vi "Transmit Messages with Rate-based Schedule.vi"() -> ()   [LabVIEW 2023]
doc: "This program opens the specified card, builds a transmit schedule \nusing transmit interval information in the channel configuration file,\nand then transmits the messages with changing data."
uses:
  <instrlib>/BTICardLib/Private/Initialize By Card Number and Core Number.vi
  <instrlib>/BTICardLib/Private/Configure Core From XML.vi
  <instrlib>/BTI429Lib/Private/Tx/Configure/Configure Tx Channel From XML.vi
  <instrlib>/BTI429Lib/Private/Core/Action-Status/Start Channel.vi
  <instrlib>/BTI429Lib/Private/Utility/Get BNR Mantissa.vi
  <instrlib>/BTI429Lib/Private/Utility/Set BNR Mantissa.vi
  <instrlib>/BTI429Lib/Private/Core/Action-Status/Stop Channel.vi
  <instrlib>/BTICardLib/BTICardLV.lvlib
  <instrlib>/BTI429Lib/BTI429LV.lvlib
panel:
  out "Core Xml Path":path
  out "Channel Xml Path":path
  in  "Card number":i32
  in  "Channel number":i32
  in  "Core number":i32
  in  "Core Configuration XML file name":string="Core Config.xml"
  in  "Channel Configuration XML file name":string="Channel Config.xml"
  out "error out":errorcluster
  in  "stop":bool
  out "Data 1(MyLabel1)":u32 format="%.0b"
  out "Data 2(MyLabel2)":u32 format="%.0b"
  out "Data 3(MyLabel3)":u32 format="%.0b"
  # "ARINC 429: Transmit Messages with Rate-based Schedule"
  # "©2016 Astronics Ballard Technology"
  # "This program opens the specified card, builds a transmit schedule \nusing transmit interval information in the channel configuration file,\nand then transmits the messages with changing data."
  # "Always Stop the card\nand Close the card when\ndone. Otherwise, the hardware\ncontinues to operate."
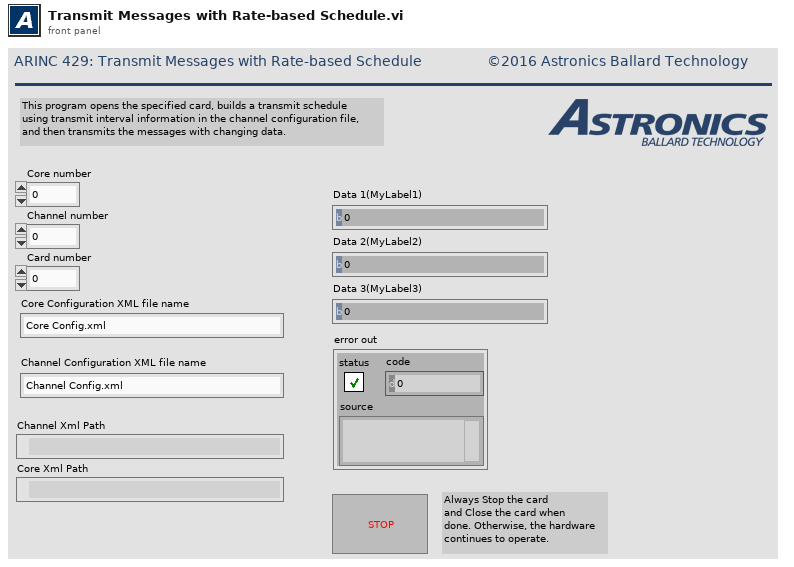
[diagram p1: front panel]
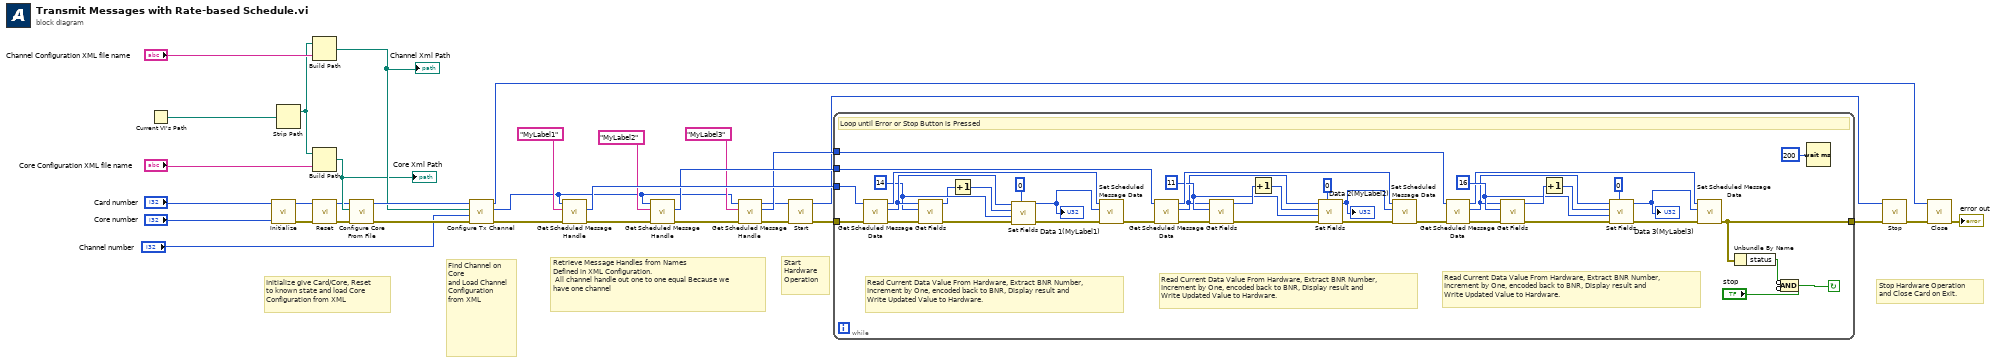
[diagram p0: block diagram]
diagram:
  # "Stop Hardware Operation\nand Close Card on Exit."
  # "Start Hardware\nOperation"
  # "Retrieve Message Handles from Names\nDefined in XML Configuration. \n All channel handle out one to one equal Because we have one channel"
  # "Find Channel on Core\nand Load Channel Configuration\nfrom XML"
  # "Initialize give Card/Core, Reset\nto known state and load Core\nConfiguration from XML"
  n1 = Current VI's Path() -> (path=w13:path)
  n2 = call-poly <instrlib>:"Initialize.vi"("core number"="Core number", "card number"="Card number") -> ("error out"=w6:errorcluster, "core handle out"=w7:u64)  [unwired: 8 in]
  n3 = Strip Path(path=w13) -> (stripped path=w10:path)  [unwired: 1 out]
  n4 = Build Path(base path=w10, name or relative path="Channel Configuration XML file name") -> (appended path=w12:path)
  "Channel Xml Path" <- w12
  n5 = Build Path(base path=w10, name or relative path="Core Configuration XML file name") -> (appended path=w8:path)
  "Core Xml Path" <- w8
  n6 = call <instrlib>:"Reset.vi"("error in (no error)"=w6, "core handle in"=w7) -> ("error out"=w4:errorcluster, "core handle out"=w5:u64)  [unwired: 8 in]
  n7 = call-poly <instrlib>:"Configure Core From File.vi"("error in (no error)"=w4, "configuration file path"=w8, "core handle in"=w5) -> ("error out"=w19:errorcluster, "core handle out"=w18:u64)  [unwired: 7 in]
  n8 = call-poly <instrlib>:"Configure Tx Channel.vi"("error in (no error)"=w19, "channel number in"="Channel number", "configuration file path"=w12, "core handle in"=w18) -> ("error out"=w33:errorcluster, "channel handle out"=w21:u64, "core handle out"=w20:u64)  [unwired: 5 in]
  n9 = call <instrlib>:"Get Scheduled Message Handle.vi"("error in (no error)"=w33, "message name"="MyLabel1" ("msgname"), "channel handle in"=w21) -> ("error out"=w28:errorcluster, "message handle out"=w31:u64)  [unwired: 6 in, 1 out]
  n10 = call <instrlib>:"Get Scheduled Message Handle.vi"("error in (no error)"=w28, "message name"="MyLabel2" ("msgname"), "channel handle in"=w21) -> ("error out"=w27:errorcluster, "message handle out"=w30:u64)  [unwired: 6 in, 1 out]
  n11 = call <instrlib>:"Get Scheduled Message Handle.vi"("error in (no error)"=w27, "message name"="MyLabel3" ("msgname"), "channel handle in"=w21) -> ("error out"=w26:errorcluster, "message handle out"=w29:u64, "channel handle out"=w15:u64)  [unwired: 6 in]
  n12 = call-poly <instrlib>:"Start.vi"("error in (no error)"=w26, "channel handle in"=w15) -> ("error out"=w32:errorcluster, "channel handle out"=w17:u64)  [unwired: 8 in]
  n13 = while {
    tunnel: [w48] -> w16
    tunnel: w29 -> [w51]
    tunnel: w30 -> [w62]
    tunnel: w32 -> [w70]
    tunnel: w31 -> [w61]
    stop <- w72 continue-if-true
    w46 = u16 16
    w47 = u16 11
    w39 = u16 14
    # "Read Current Data Value From Hardware, Extract BNR Number,\nIncrement by One, encoded back to BNR, Display result and\nWrite Updated Value to Hardware."
    # "Read Current Data Value From Hardware, Extract BNR Number,\nIncrement by One, encoded back to BNR, Display result and\nWrite Updated Value to Hardware."
    # "Read Current Data Value From Hardware, Extract BNR Number,\nIncrement by One, encoded back to BNR, Display result and\nWrite Updated Value to Hardware."
    # "Loop until Error or Stop Button is Pressed"
    n14 = call <instrlib>:"Get Scheduled Message Data.vi"("error in (no error)"=w70, "message handle in"=w61) -> ("error out"=w71:errorcluster, "value"=w41:u32, "message handle out"=w69:u64)  [unwired: 7 in]
    n15 = call-poly <instrlib>:"Get Fields.vi"("error in (no error)"=w71, "significant digits"=w39, "message"=w41) -> ("error out"=w40:errorcluster, "mantissa out"=w36:u32)  [unwired: 7 in]
    n16 = Increment(x=w36) -> (x+1=w35:u32)
    n17 = call-poly <instrlib>:"Set Fields.vi"("twos"=u16 0, "error in (no error)"=w40, "significant bits"=w39, "value"=w35, "message"=w41) -> ("error out"=w37:errorcluster, "message out"=w34:u32)  [unwired: 5 in]
    "Data 1(MyLabel1)" <- w34
    n18 = call <instrlib>:"Set Scheduled Message Data.vi"("error in (no error)"=w37, "value"=w34, "message handle in"=w69) -> ("error out"=w58:errorcluster)  [unwired: 7 in, 1 out]
    n19 = call <instrlib>:"Get Scheduled Message Data.vi"("error in (no error)"=w58, "message handle in"=w62) -> ("error out"=w68:errorcluster, "value"=w43:u32, "message handle out"=w63:u64)  [unwired: 7 in]
    n20 = call-poly <instrlib>:"Get Fields.vi"("error in (no error)"=w68, "significant digits"=w47, "message"=w43) -> ("error out"=w67:errorcluster, "mantissa out"=w65:u32)  [unwired: 7 in]
    n21 = Increment(x=w65) -> (x+1=w64:u32)
    n22 = call-poly <instrlib>:"Set Fields.vi"("twos"=u16 0, "error in (no error)"=w67, "significant bits"=w47, "value"=w64, "message"=w43) -> ("error out"=w66:errorcluster, "message out"=w59:u32)  [unwired: 5 in]
    "Data 2(MyLabel2)" <- w59
    n23 = call <instrlib>:"Set Scheduled Message Data.vi"("error in (no error)"=w66, "value"=w59, "message handle in"=w63) -> ("error out"=w52:errorcluster)  [unwired: 7 in, 1 out]
    n24 = call <instrlib>:"Get Scheduled Message Data.vi"("error in (no error)"=w52, "message handle in"=w51) -> ("error out"=w57:errorcluster, "value"=w44:u32, "message handle out"=w45:u64)  [unwired: 7 in]
    n25 = call-poly <instrlib>:"Get Fields.vi"("error in (no error)"=w57, "significant digits"=w46, "message"=w44) -> ("error out"=w56:errorcluster, "mantissa out"=w54:u32)  [unwired: 7 in]
    n26 = Increment(x=w54) -> (x+1=w53:u32)
    n27 = call-poly <instrlib>:"Set Fields.vi"("twos"=u16 0, "error in (no error)"=w56, "significant bits"=w46, "value"=w53, "message"=w44) -> ("error out"=w55:errorcluster, "message out"=w50:u32)  [unwired: 5 in]
    "Data 3(MyLabel3)" <- w50
    n28 = call <instrlib>:"Set Scheduled Message Data.vi"("error in (no error)"=w55, "value"=w50, "message handle in"=w45) -> ("error out"=w48:errorcluster)  [unwired: 7 in, 1 out]
    n29 = Unbundle By Name(w48) -> ("status"=w73:bool)
    n30 = Compound Arithmetic op=AND(invert w73, invert "stop") -> (w72:bool)
    n31 = Wait (ms)(milliseconds to wait=u32 200) -> ()  [unwired: 1 out]
  }
  n32 = call-poly <instrlib>:"Stop.vi"("error in (no error)"=w16, "channel handle in"=w17) -> ("error out"=w14:errorcluster)  [unwired: 8 in, 1 out]
  n33 = call <instrlib>:"Close.vi"("error in (no error)"=w14, "core handle in"=w20) -> ("error out"=→"error out":errorcluster)  [unwired: 8 in, 1 out]
